vi "_Spark Single LC Driver.vi"   [LabVIEW 2012]
uses:
  C:/Users/Min/Projects/SVN/PEI Sniffer 900/LCDriver/Ionics.Spark.Driver.dll
  Ionics.Spark.Driver.dll
  Type/_Log Command.ctl
  _Global LC Driver.vi
types:
  T1 = cluster{"new reference":refnum<k24>, "Initialized":bool}
  T2 = typedef "_Log Command.ctl" = enum16{"No Command", "Open", "Read", "Write", "Close", "Check Size"}
  T3 = typedef "_LC Command.ctl" = enum16{"No Command", "Initialize", "Get Configuration", "Get Status", "Get LC Method Contents", "Oven OnOff", "Pump OnOFF", "Rinse Autosampler", "Run Sample", "Set EnvParameters", "Set Method", "Start Equilibration", "Stop Run", "Get LastError", "Clear Error", "Close"}
  T4 = cluster{"PlatePosition":u8, "SampleColumn":u8, "TrayType":u8}
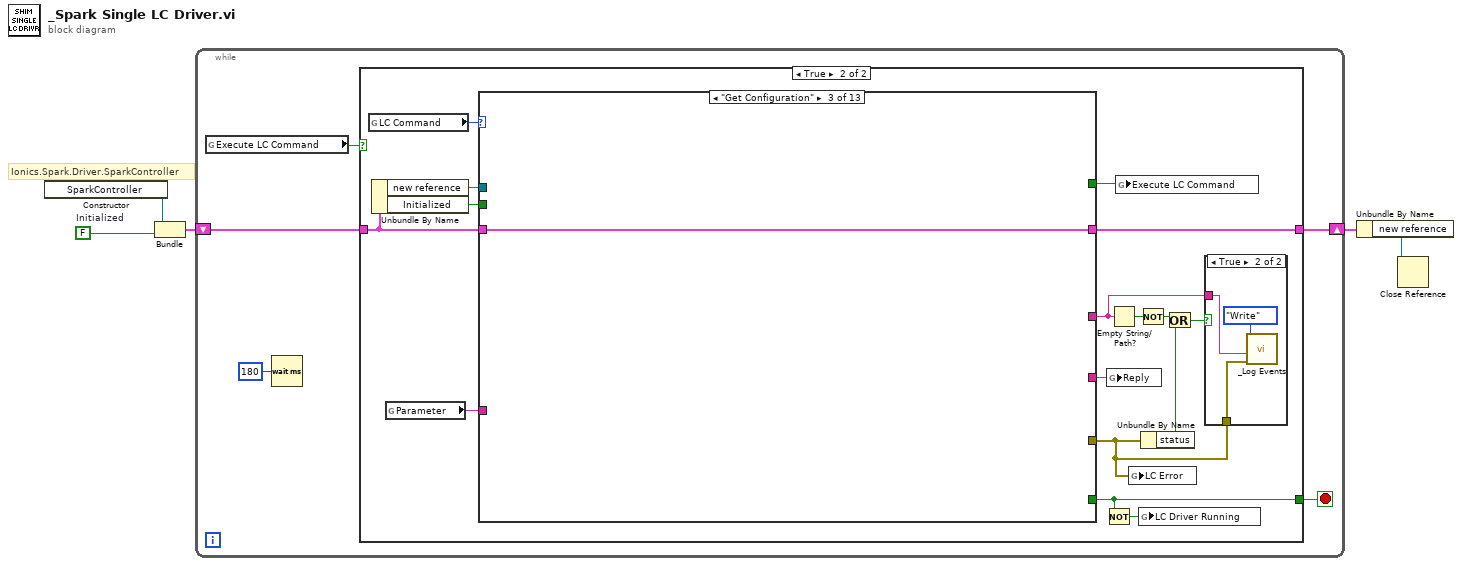
[diagram p0: block diagram]
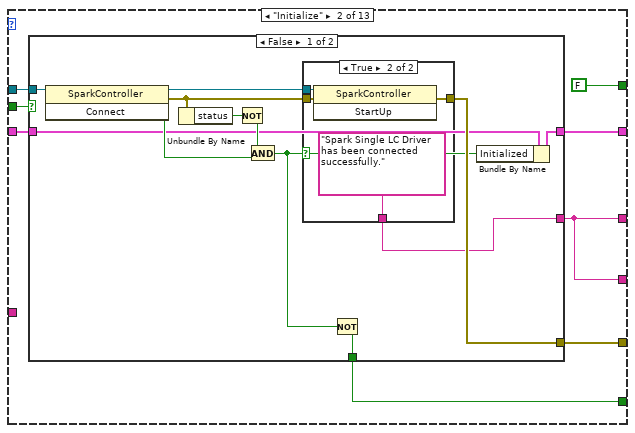
[diagram p5: hidden frame]
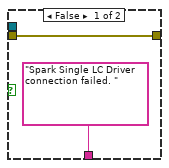
[diagram p6: hidden frame]
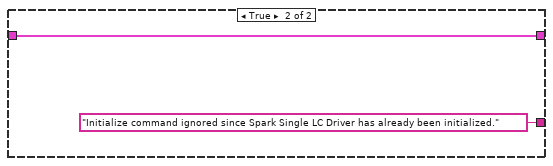
[diagram p7: hidden frame]
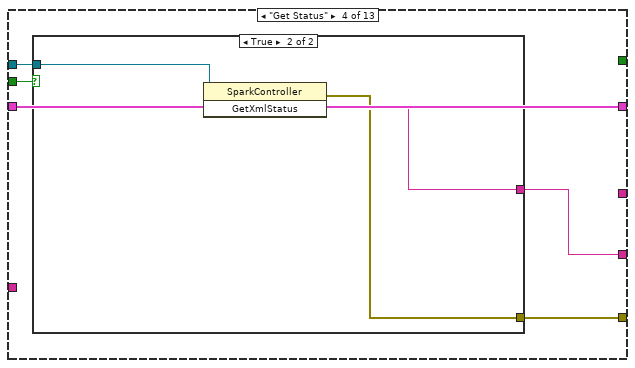
[diagram p8: hidden frame]
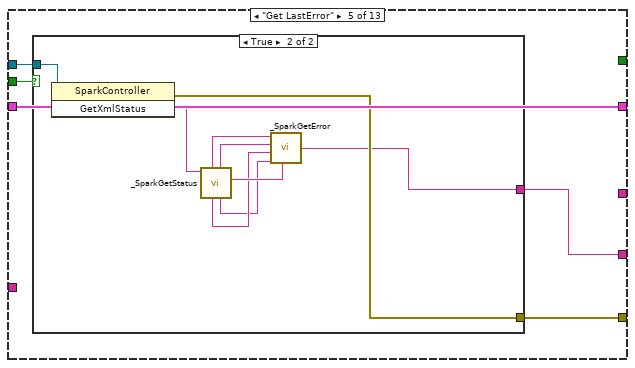
[diagram p10: hidden frame]
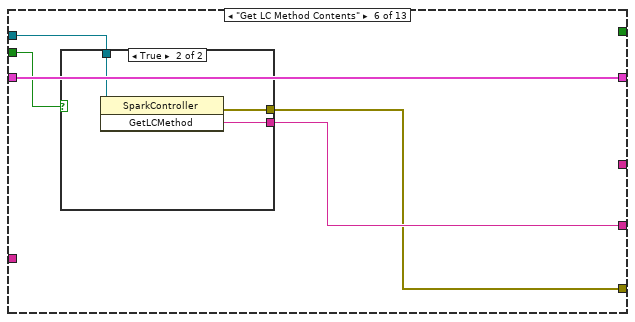
[diagram p12: hidden frame]
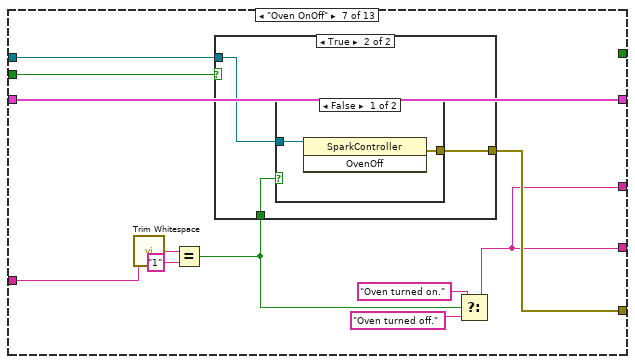
[diagram p14: hidden frame]
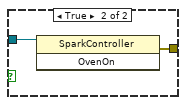
[diagram p16: hidden frame]
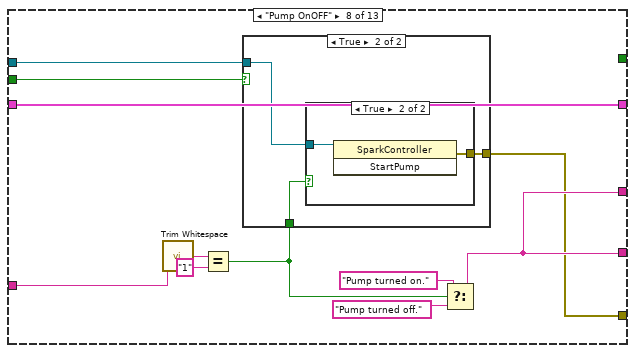
[diagram p17: hidden frame]
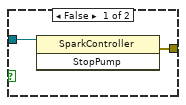
[diagram p19: hidden frame]
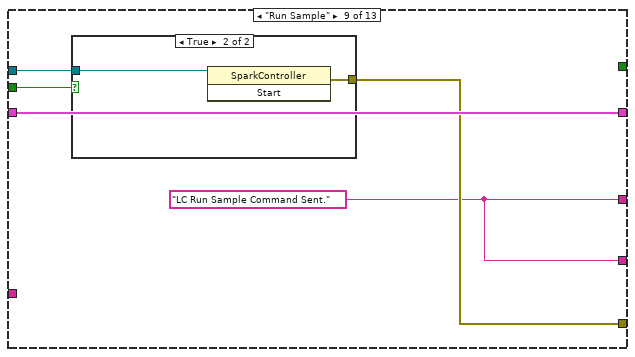
[diagram p20: hidden frame]
diagram:
  w5 = FALSE  # Initialized
  # "Ionics.Spark.Driver.SparkController"
  n1 = constructor class="SparkController" ("Controller")() -> (reference out=w3:refnum<k24>)  [unwired: 3 in, 2 out]
  n2 = Bundle("new reference"=w3, "Initialized"=w5) -> (w4:T1)  [unwired: 1 in]
  n3 = while {
    shift-right: [w10] -> w2
    shift-left: w4 -> [w9]
    stop <- w7 stop-if-true
    n4 = global read "_Global LC Driver.vi" "Execute LC Command"() -> (w6:bool)
    n5 = Wait (ms)(milliseconds to wait=u32 180) -> ()  [unwired: 1 out]
    n6 = case shown="True" w6 {
      tunnel: [w11 w19] -> w10
      tunnel: w9 -> [w11 w14]
      tunnel: [_ w20] -> w7
      frame False {
      }
      frame True {
        n7 = global read "_Global LC Driver.vi" "LC Command"() -> (w18:T3)
        n8 = Unbundle By Name(w14) -> ("new reference"=w13:refnum<k24>, "Initialized"=w12:bool)
        n9 = global read "_Global LC Driver.vi" "Parameter"() -> (w15:string)
        n10 = case shown="\"Get Configuration\"" w18 {
          tunnel: [w31 w39 w60 w65 w73 w87 w99 w119 w131 w140 w155 w162 w170] -> w19
          tunnel: w14 -> [w31 w38 w60 w65 w73 w87 w99 w119 w131 w140 w155 w162 w171]
          tunnel: [_ w37 _ w61 w69 w84 w98 w109 w130 w139 w154 w161 w169] -> w22
          tunnel: [_ w32 _ _ _ _ w92 w111 w127 w138 w151 w158 w165] -> w23
          tunnel: w13 -> [_ w35 _ w63 w71 w86 w93 w112 w128 w135 w152 w159 w167]
          tunnel: w12 -> [_ w36 _ w64 w72 w83 w94 w113 w129 w136 w153 w160 w168]
          tunnel: [_ w34 _ _ _ _ _ _ _ _ _ _ TRUE] -> w20
          tunnel: [_ FALSE _ _ _ _ _ _ _ _ _ _ _] -> w17
          tunnel: [_ w32 _ w62 w70 w85 w92 w111 w127 w137 w151 w158 w165] -> w16
          tunnel: w15 -> [_ _ _ _ _ _ w91 w110 _ w134 _ _ _]
          frame "No Command", Default {
          }
          frame "Initialize" {
            n11 = case shown="False" w36 {
              tunnel: [w51 _] -> w37
              tunnel: [w42 w59] -> w39
              tunnel: w38 -> [w43 w59]
              tunnel: [w45 "Initialize command ignored since Spark Single LC Driver has already been initialized." ("Event")] -> w32
              tunnel: w35 -> [w44 _]
              tunnel: [w41 _] -> w34
              frame False {
                n12 = invoke class="SparkController" method="Connect"(reference=w44) -> (reference out=w50:refnum<k24>, error out=w46:errorcluster, "Connect"=w48:bool)  [unwired: 2 in]
                n13 = Unbundle By Name(w46) -> ("status"=w49:bool)
                n14 = Not(x=w49) -> (.not. x?=w47:bool)
                n15 = And(x=w47, y=w48) -> (x .and. y?=w40:bool)
                n16 = case shown="True" w40 {
                  tunnel: w50 -> [_ w57]
                  tunnel: [w53 w54] -> w51
                  tunnel: w46 -> [w53 w56]
                  tunnel: ["Spark Single LC Driver connection failed. " ("Event") "Spark Single LC Driver has been connected successfully." ("Event")] -> w45
                  frame False {
                  }
                  frame True {
                    n17 = invoke class="SparkController" method="StartUp"(reference=w57, error in=w56) -> (error out=w54:errorcluster)  [unwired: 1 in, 2 out]
                  }
                }
                n18 = Not(x=w40) -> (.not. x?=w41:bool)
                n19 = Bundle By Name(cluster=w43, "Initialized"=w40) -> (w42:T1)
              }
              frame True {
              }
            }
          }
          frame "Get Configuration" {
          }
          frame "Get Status" {
            n20 = case shown="True" w64 {
              tunnel: w63 -> [_ w68]
              tunnel: [_ w67] -> w62
              tunnel: [_ w66] -> w61
              frame False {
              }
              frame True {
                n21 = invoke class="SparkController" method="GetXmlStatus"(reference=w68) -> (error out=w66:errorcluster, "GetXmlStatus"=w67:string)  [unwired: 2 in, 1 out]
              }
            }
          }
          frame "Get LastError" {
            n22 = case shown="True" w72 {
              tunnel: w71 -> [_ w82]
              tunnel: [_ w74] -> w70
              tunnel: [_ w81] -> w69
              frame False {
              }
              frame True {
                n23 = invoke class="SparkController" method="GetXmlStatus"(reference=w82) -> (error out=w81:errorcluster, "GetXmlStatus"=w80:string)  [unwired: 2 in, 1 out]
                n24 = call "_SparkGetStatus.vi"("SparkStatus"=w80) -> ("LCStatus"=w77:string, "PumpB Status"=w75:string, "Oven Status"=w78:string, "PumpA Status"=w76:string, "AS Status"=w79:string)  [unwired: 3 in, 3 out]
                n25 = call "_SparkGetError.vi"("AS Status"=w79, "Oven Status"=w78, "Pump 1 Status"=w76, "Pump 2 Status"=w75, "LC Status"=w77) -> ("LC Error"=w74:string)
              }
            }
          }
          frame "Get LC Method Contents" {
            n26 = case shown="True" w83 {
              tunnel: w86 -> [_ w90]
              tunnel: [_ w89] -> w85
              tunnel: [_ w88] -> w84
              frame False {
              }
              frame True {
                n27 = invoke class="SparkController" method="GetLCMethod"(reference=w90) -> (error out=w88:errorcluster, "GetLCMethod"=w89:string)  [unwired: 2 in, 1 out]
              }
            }
          }
          frame "Oven OnOff" {
            n28 = call <vilib>:"Trim Whitespace.vi"("string"=w91) -> ("trimmed string"=w101:string)  [unwired: 1 in]
            n29 = Equal?(x=w101, y="1") -> (x = y?=w95:bool)
            n30 = case shown="True" w94 {
              tunnel: w95 -> [_ w103]
              tunnel: [_ w104] -> w98
              tunnel: w93 -> [_ w102]
              frame False {
              }
              frame True {
                n31 = case shown="False" w103 {
                  tunnel: w102 -> [w106 w108]
                  tunnel: [w105 w107] -> w104
                  frame False {
                    n32 = invoke class="SparkController" method="OvenOff"(reference=w106) -> (error out=w105:errorcluster)  [unwired: 2 in, 2 out]
                  }
                  frame True {
                    n33 = invoke class="SparkController" method="OvenOn"(reference=w108) -> (error out=w107:errorcluster)  [unwired: 2 in, 2 out]
                  }
                }
              }
            }
            n34 = Select(t="Oven turned on." ("y"), s=w95, f="Oven turned off." ("y")) -> (s? t:f=w92:string)
          }
          frame "Pump OnOFF" {
            n35 = call <vilib>:"Trim Whitespace.vi"("string"=w110) -> ("trimmed string"=w118:string)  [unwired: 1 in]
            n36 = Equal?(x=w118, y="1") -> (x = y?=w116:bool)
            n37 = case shown="True" w113 {
              tunnel: w116 -> [_ w122]
              tunnel: w112 -> [_ w121]
              tunnel: [_ w120] -> w109
              frame False {
              }
              frame True {
                n38 = case shown="True" w122 {
                  tunnel: w121 -> [w124 w126]
                  tunnel: [w123 w125] -> w120
                  frame False {
                    n39 = invoke class="SparkController" method="StopPump"(reference=w124) -> (error out=w123:errorcluster)  [unwired: 2 in, 2 out]
                  }
                  frame True {
                    n40 = invoke class="SparkController" method="StartPump"(reference=w126) -> (error out=w125:errorcluster)  [unwired: 2 in, 2 out]
                  }
                }
              }
            }
            n41 = Select(t="Pump turned on." ("y"), s=w116, f="Pump turned off." ("y")) -> (s? t:f=w111:string)
          }
          frame "Run Sample" {
            w127 = "LC Run Sample Command Sent." ("y")
            n42 = case shown="True" w129 {
              tunnel: [_ w133] -> w130
              tunnel: w128 -> [_ w132]
              frame False {
              }
              frame True {
                n43 = invoke class="SparkController" method="Start"(reference=w132) -> (error out=w133:errorcluster)  [unwired: 2 in, 2 out]
              }
            }
          }
          frame "Set Method" {
            n44 = case shown="True" w136 {
              tunnel: [_ w148] -> w139
              tunnel: [_ w149] -> w138
              tunnel: [_ w149] -> w137
              tunnel: w135 -> [_ w145]
              tunnel: w134 -> [_ w141]
              frame False {
              }
              frame True {
                n45 = global read "_Global LC Driver.vi" "InjectionVolume"() -> (w144:dbl)
                n46 = global read "_Global LC Driver.vi" "VialNumber"() -> (w143:i16)
                n47 = global read "_Global LC Driver.vi" "SparkParameters"() -> (w147:T4)
                n48 = Unbundle By Name(w147) -> ("PlatePosition"=w142:u8, "TrayType"=w146:u8)  [unwired: 1 out]
                n49 = Format Into String(format string="LC Set Method Command Sent: File=%s; Rack=%d; Plate=%d; Vial=%d; Volume=%f.", w141, w146, w142, w143, w144) -> (resulting string=w149:string)  [unwired: 2 in, 1 out]
                n50 = invoke class="SparkController" method="Prepare"(reference=w145, "methodFile"=w141, "platePosition"=w142, "sampleVial"=w143, "injectionVolume"=w144) -> (error out=w148:errorcluster)  [unwired: 2 in, 6 out]
              }
            }
          }
          frame "Stop Run" {
            w151 = "LC Stop Run Command Sent." ("y")
            n51 = case shown="True" w153 {
              tunnel: w152 -> [_ w157]
              tunnel: [_ w156] -> w154
              frame False {
              }
              frame True {
                n52 = invoke class="SparkController" method="Abort"(reference=w157) -> (error out=w156:errorcluster)  [unwired: 2 in, 2 out]
              }
            }
          }
          frame "Clear Error" {
            w158 = "LC Clear Error Command Sent." ("y")
            n53 = case shown="True" w160 {
              tunnel: w159 -> [_ w164]
              tunnel: [_ w163] -> w161
              frame False {
              }
              frame True {
                n54 = invoke class="SparkController" method="ResetAllErrors"(reference=w164) -> (error out=w163:errorcluster)  [unwired: 2 in, 2 out]
              }
            }
          }
          frame "Close" {
            w165 = "Spark Single LC Driver is disconnected." ("Event")
            n55 = case shown="True" w168 {
              tunnel: [_ w174] -> w169
              tunnel: w167 -> [_ w173]
              frame False {
              }
              frame True {
                n56 = invoke class="SparkController" method="Shutdown"(reference=w173) -> (reference out=w175:refnum<k24>)  [unwired: 2 in, 2 out]
                n57 = stacked-sequence {
                  tunnel: w175 -> [_ w178]
                  tunnel: [_ w177] -> w174
                  frame #0 {
                    n58 = Wait (ms)(milliseconds to wait=u32 1000) -> ()  [unwired: 1 out]
                  }
                  frame #1 {
                    n59 = invoke class="SparkController" method="Disconnect"(reference=w178) -> (error out=w177:errorcluster)  [unwired: 2 in, 2 out]
                  }
                }
              }
            }
            n60 = Bundle By Name(cluster=w171, "Initialized"=FALSE) -> (w170:T1)
          }
        }
        n61 = Not(x=w20) -> (.not. x?=w21:bool)
        n62 = global write "_Global LC Driver.vi" "Reply"(w16) -> ()
        n63 = Empty String/Path?(string/path=w23) -> (empty?=w27:bool)
        n64 = global write "_Global LC Driver.vi" "Execute LC Command"(w17) -> ()
        n65 = global write "_Global LC Driver.vi" "LC Error"(w22) -> ()
        n66 = Not(x=w27) -> (.not. x?=w26:bool)
        n67 = global write "_Global LC Driver.vi" "LC Driver Running"(w21) -> ()
        n68 = Unbundle By Name(w22) -> ("status"=w25:bool)
        n69 = Or(x=w26, y=w25) -> (x .or. y?=w24:bool)
        n70 = case shown="True" w24 {
          tunnel: w22 -> [_ w28]
          tunnel: w23 -> [_ w29]
          frame False {
          }
          frame True {
            n71 = call "_Log Events.vi"("error in (no error)"=w28, "Event"=w29, "Log Command"=_Log_Command."Write") -> ()  [unwired: 1 in, 5 out]
          }
        }
      }
    }
  }
  n72 = Unbundle By Name(w2) -> ("new reference"=w1:refnum<k24>)
  n73 = Close Reference(reference=w1) -> ()  [unwired: 1 in, 1 out]
